vi "Read XML HW Configuration File_Parse Channels.vi"(8 "error in (no error)":errorcluster, 11 "channel429":refnum<k24>[](array[refnum])) -> (0 "error out":errorcluster, 3 "Array":T1[](array[typedef]) {"speed" items=["Auto", "Low", "High"]; "Labels"."scheduleBuildUnit" items=["Millisecond", "Microsecond"]})   [LabVIEW 2020]
doc: "This VI parses the XML HW DB."
uses:
  Controls/Ballard_Channel.ctl
  Controls/Ballard_Label.ctl
  Controls/Ballard_Word.ctl
  Controls/ARINCParam.ctl
  Shared/Controls and Global/TransferType.ctl
  Controls/Channel_direction.ctl
  Controls/Channel Speed.ctl
  C:/Users/NI/Desktop/GIT/Ballard-Arinc-429-Custom-Device/Source/System Explorer/SubVIs/Parse XML Ballard/Ballard_BTI_XML_Deserializer.dll
  Ballard_BTI_XML_Deserializer.dll
  Ballard Arinc-429 System Explorer.lvlib
  Shared/Ballard Arinc-429 Shared.lvlib
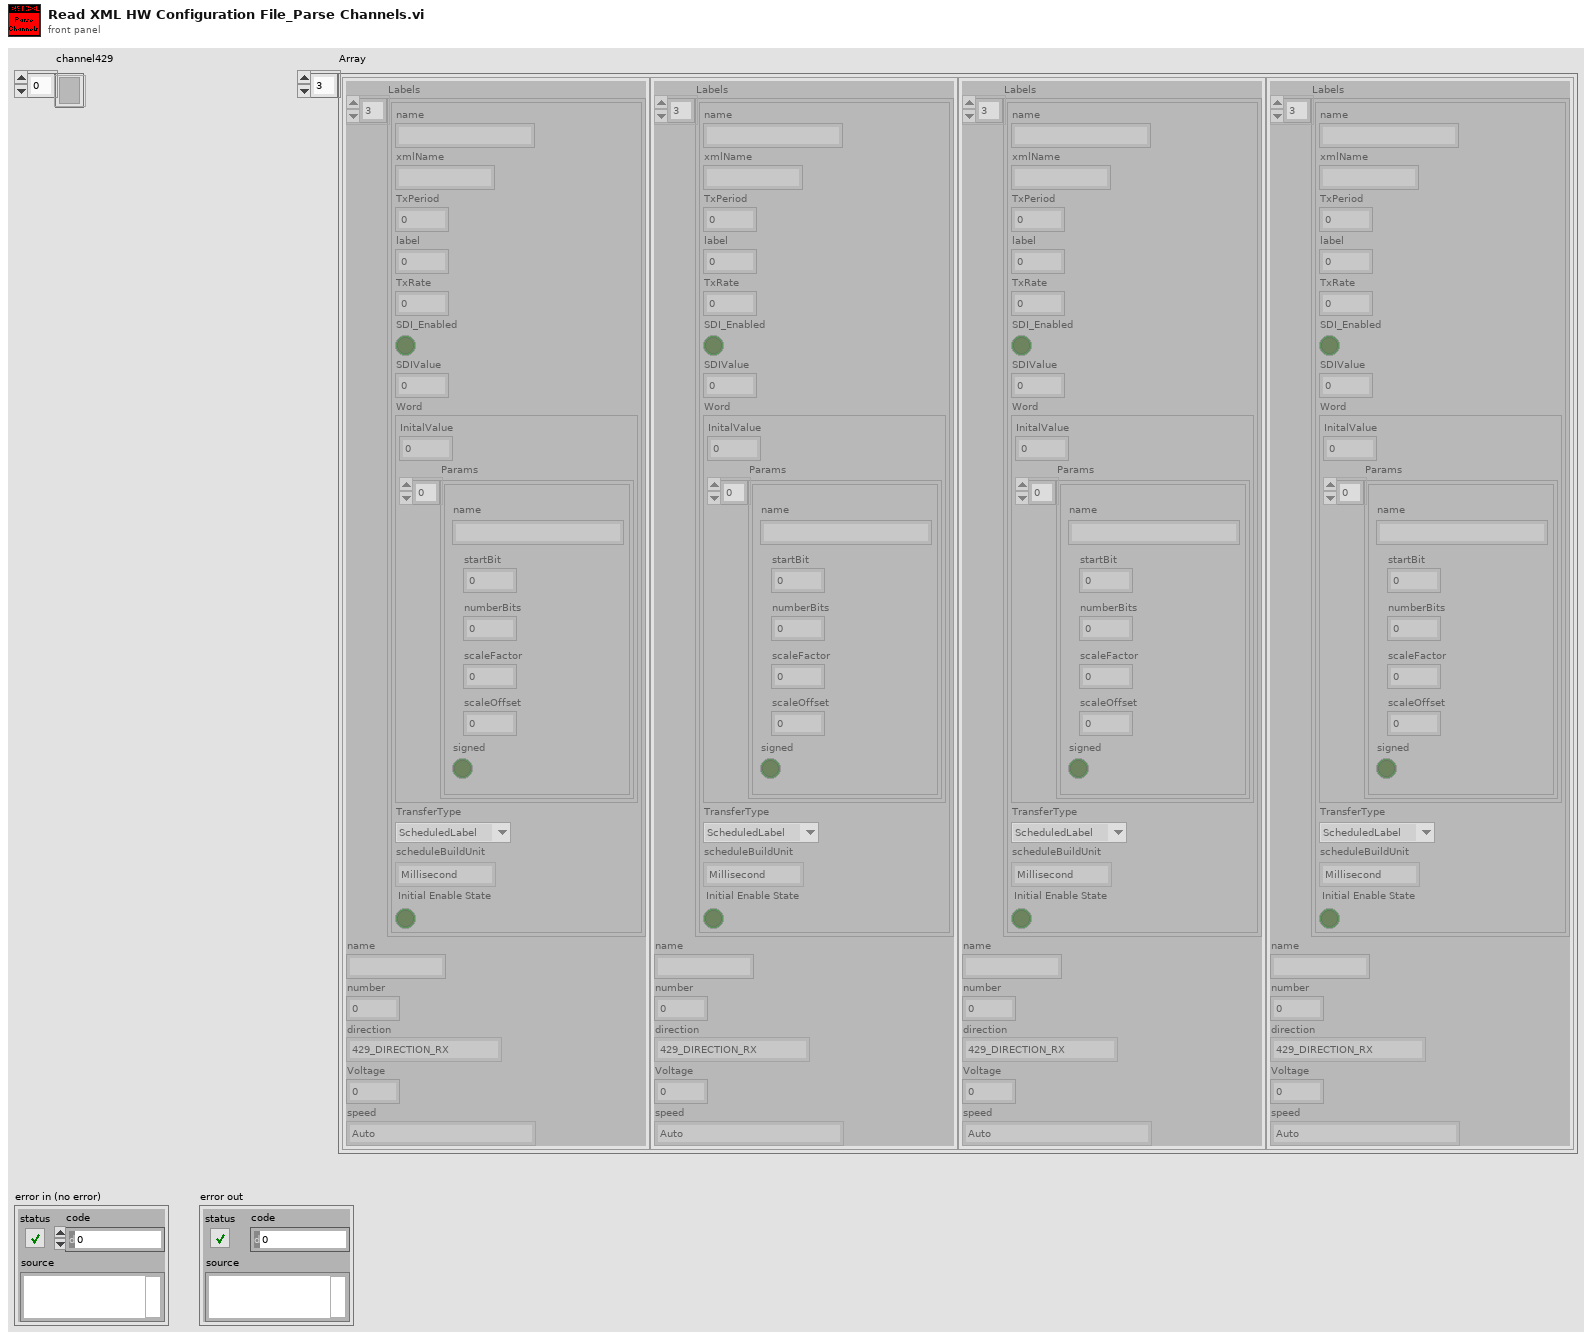
[diagram p1: front panel]
types:
  T1 = typedef "Ballard Arinc-429 System Explorer.lvlib/Ballard_Channel.ctl" = cluster{"Labels":T2[], "name":string, "number":u8, "direction":T6, "Voltage":dbl, "speed":T7}
  T2 = typedef "Ballard Arinc-429 System Explorer.lvlib/Ballard_Label.ctl" = cluster{"name":string, "xmlName":string, "TxPeriod":u32, "label":u32, "TxRate":dbl, "SDI_Enabled":bool, "SDIValue":u8, "Word":T3, "TransferType":T5, "scheduleBuildUnit":i32, "Initial Enable State":bool}
  T3 = typedef "Ballard Arinc-429 System Explorer.lvlib/Ballard_Word.ctl" = cluster{"InitalValue":u32, "Params":T4[]}
  T4 = typedef "Ballard Arinc-429 System Explorer.lvlib/ARINCParam.ctl" = cluster{"name":string, "startBit":i32, "numberBits":i32, "scaleFactor":dbl, "scaleOffset":dbl, "signed":bool}
  T5 = typedef "Ballard Arinc-429 Shared.lvlib/TransferType.ctl" = enum16{"ScheduledLabel", "Acyclic", "Block", "Strobe"}
  T6 = typedef "Ballard Arinc-429 System Explorer.lvlib/Channel_direction.ctl" = enum16{"429_DIRECTION_RX", "429_DIRECTION_TX"}
  T7 = typedef "Ballard Arinc-429 System Explorer.lvlib/Channel Speed.ctl" = i32
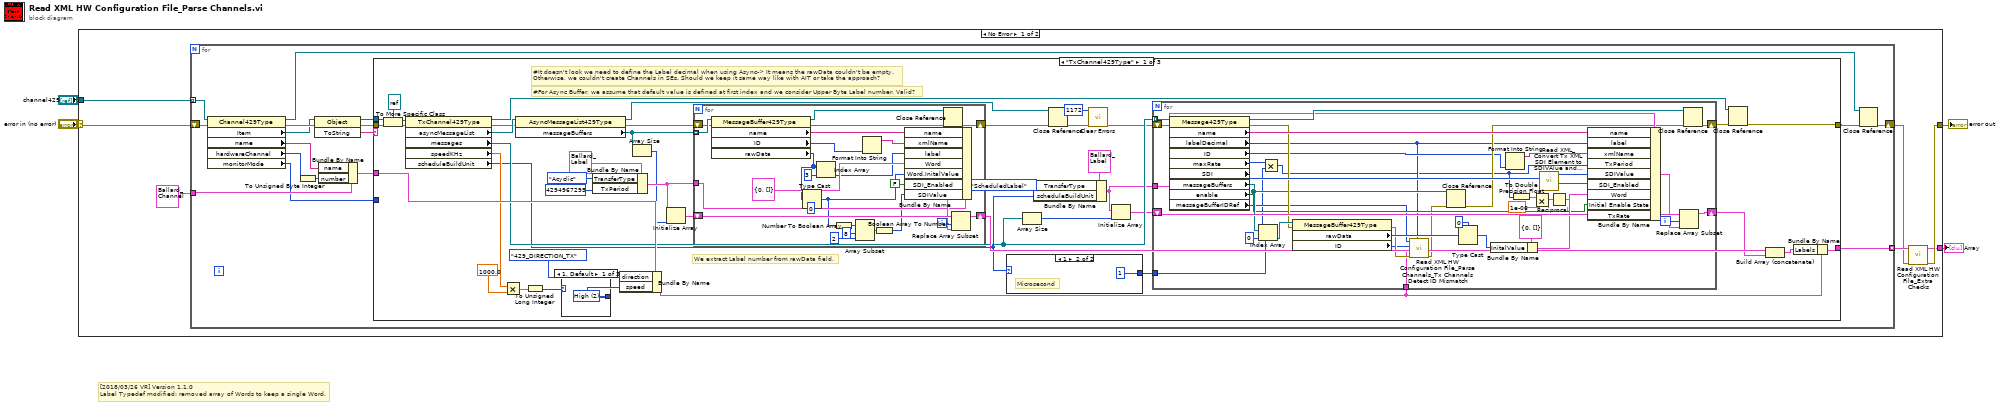
[diagram p0: block diagram]
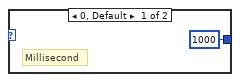
[diagram p2: hidden frame]
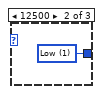
[diagram p3: hidden frame]
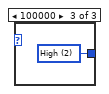
[diagram p4: hidden frame]
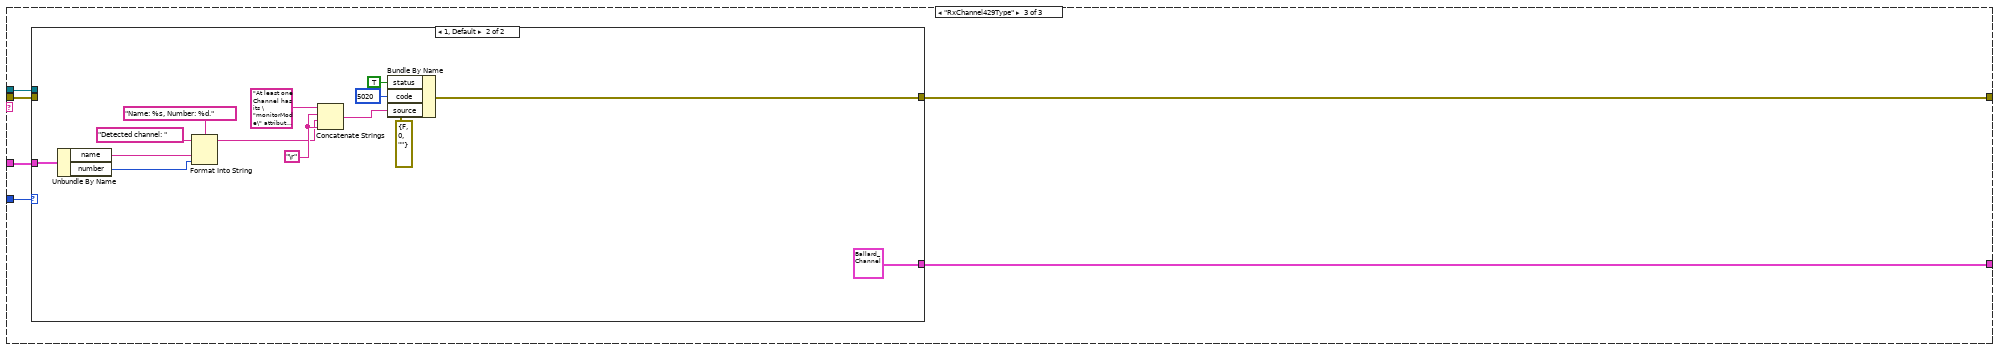
[diagram p6: hidden frame]
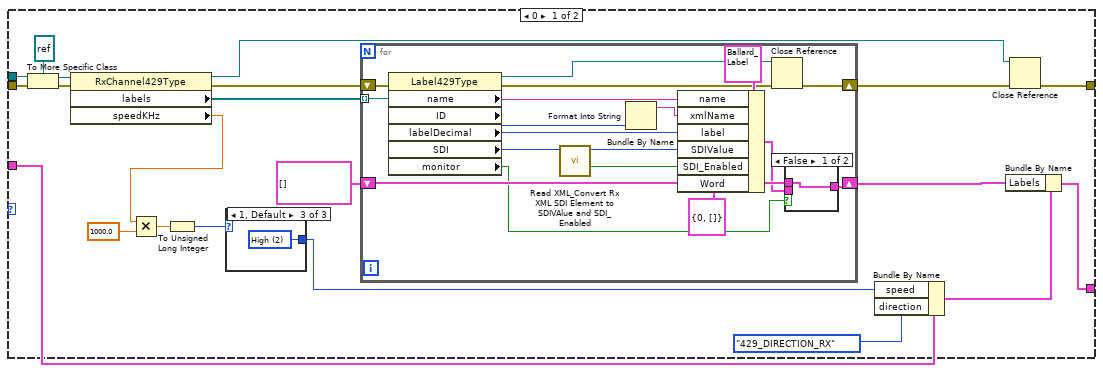
[diagram p7: hidden frame]
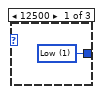
[diagram p8: hidden frame]
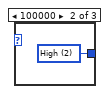
[diagram p9: hidden frame]
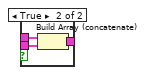
[diagram p10: hidden frame]
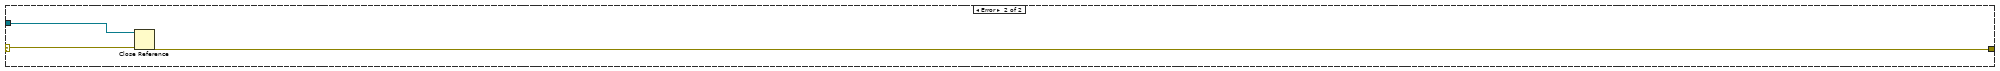
[diagram p11: hidden frame]
diagram:
  # "[2018/03/26 VR] Version 1.1.0\nLabel Typedef modified: removed array of Words to keep a single Word."
  n1 = case shown="No Error" "error in (no error)" {
    selector: "error in (no error)" -> [w9 w210]
    tunnel: [w5 _] -> w4
    tunnel: [w6 w209] -> w3
    tunnel: "channel429" -> [w10 w211]
    frame No Error {
      n2 = for {
        tunnel: w10 -> [w28] mode=indexing
        shift-right: [w16] -> w7
        shift-left: w9 -> [w25]
        tunnel: T1 {"Labels"=[], "name"="", "number"=0, "direction"=enum."429_DIRECTION_RX", "Voltage"=0.0, "speed"=0} ("channel") -> [w21]
        tunnel: [w12] -> w8 mode=indexing
        n3 = property class="Channel429Type"(reference=w28, error in=w25) -> (reference out=w15:refnum<k24>, error out=w24:errorcluster, "Item"=w22:refnum<k24>, "name"=w20:string, "hardwareChannel"=w19:i32, "monitorMode"=w14:i32)
        n4 = To Unsigned Byte Integer(number=w19) -> (unsigned 8bit integer=w18:u8)
        n5 = invoke class="Object" method="ToString"(reference=w22, error in=w24) -> (reference out=w26:refnum<k24>, error out=w23:errorcluster, "ToString"=w27:string)  [unwired: 1 in]
        n6 = Bundle By Name(cluster=w21, "name"=w20, "number"=w18) -> (w17:T1)
        n7 = case shown="\"TxChannel429Type\"" w27 {
          tunnel: w26 -> [w71 _ w148]
          tunnel: w23 -> [w70 w142 w147]
          tunnel: [w58 w142 w144] -> w13
          tunnel: w17 -> [w56 w141 w145]
          tunnel: [w45 w141 w146] -> w12
          tunnel: w14 -> [_ _ w143]
          frame "TxChannel429Type" {
            # "We extract Label number from rawData field."
            # "#For Async Buffer, we assume that default value is defined at first index and we consider Upper Byte Label number. Valid?"
            # "#It doesn't look we need to define the Label decimal when using Async-> It means the rawData couldn't be empty.\nOtherwise, we couldn't create Channels in SEs. Should we keep it same way like with AIT or take the approach?"
            n8 = To More Specific Class(target class=refnum<k24> refnum, reference=w71, error in=w70) -> (specific class reference=w67:refnum<k24>, error out=w68:errorcluster)
            n9 = property class="TxChannel429Type"(reference=w67, error in=w68) -> (reference out=w59:refnum<k24>, error out=w65:errorcluster, "asyncMessageList"=w66:refnum<k24>, "messages"=w43:refnum<k24>[], "speedKHz"=w38:dbl, "scheduleBuildUnit"=w30:i32)
            n10 = Multiply(x=w38, y=1000.0) -> (x*y=w39:dbl)
            n11 = property class="AsyncMessageList429Type"(reference=w66, error in=w65) -> (reference out=w61:refnum<k24>, error out=w64:errorcluster, "messageBuffers"=w52:refnum<k24>[])
            n12 = To Unsigned Long Integer(number=w39) -> (unsigned 32bit integer=w36:u32)
            n13 = case shown="1, Default" w36 {
              tunnel: [w74 w75 w76] -> w35
              frame 1, Default {
                w74 = T7 2 items=["Auto", "Low", "High"] ("speed")
              }
              frame 12500 {
                w75 = T7 1 items=["Auto", "Low", "High"] ("speed")
              }
              frame 100000 {
                w76 = T7 2 items=["Auto", "Low", "High"] ("speed")
              }
            }
            n14 = Bundle By Name(cluster=T2 {"name"="", "xmlName"="", "TxPeriod"=0, "label"=0, "TxRate"=0.0, "SDI_Enabled"=FALSE, "SDIValue"=0, "Word"={"InitalValue"=0, "Params"=[]}, "TransferType"=enum."ScheduledLabel", "scheduleBuildUnit"=0, "Initial Enable State"=FALSE} ("Label"), "TransferType"=TransferType."Acyclic", "TxPeriod"=u32 4294967295) -> (w53:T2)
            n15 = Bundle By Name(cluster=w56, "direction"=Channel_direction."429_DIRECTION_TX", "speed"=w35) -> (w31:T1)
            n16 = Array Size(array=w52) -> (size(s)=w51:i32)
            n17 = Initialize Array(w53, w51) -> (w50:T2[])
            n18 = for {
              tunnel: w52 -> [w140] mode=indexing
              shift-right: [w136] -> w63
              shift-left: w64 -> [w139]
              tunnel: w53 -> [w131]
              shift-right: [w134] -> w48
              shift-left: w50 -> [w135]
              i -> [w133]
              n19 = property class="MessageBuffer429Type"(reference=w140, error in=w139) -> (reference out=w137:refnum<k24>, error out=w138:errorcluster, "name"=w130:string, "ID"=w129:i32, "rawData"=w124:u8[])
              n20 = Type Cast(type=u32 0, x=w124) -> (*(type *) &x=w117:u32)
              n21 = Index Array(array=w124, index=3) -> (element=w123:u8)
              n22 = Number To Boolean Array(number=w117) -> (Boolean array=w118:bool[])
              n23 = Array Subset(array=w118, index=8, length=2) -> (w119:bool[])
              n24 = Format Into String(w129) -> (resulting string=w128:string)  [unwired: 3 in, 1 out]
              n25 = Boolean Array To Number(Boolean array=w119) -> (number=w116:u8)
              n26 = Bundle By Name(cluster=w131, "name"=w130, "xmlName"=w128, "label"=w123, "Word"=T3 {"InitalValue"=0, "Params"=[]}, "Word.InitalValue"=w117, "SDI_Enabled"=FALSE, "SDIValue"=w116) -> (w132:T2)
              n27 = Close Reference(reference=w137, error in (no error)=w138) -> (error out=w136:errorcluster)
              n28 = Replace Array Subset(array=w135, new element=w132, index=w133) -> (w134:T2[])
            }
            n29 = case shown="1" w30 {
              tunnel: [1000 1] -> w29
              frame 0, Default {
                # "Millisecond"
              }
              frame 1 {
                # "Microsecond"
              }
            }
            n30 = Array Size(array=w43) -> (size(s)=w41:i32)
            n31 = Bundle By Name(cluster=T2 {"name"="", "xmlName"="", "TxPeriod"=0, "label"=0, "TxRate"=0.0, "SDI_Enabled"=FALSE, "SDIValue"=0, "Word"={"InitalValue"=0, "Params"=[]}, "TransferType"=enum."ScheduledLabel", "scheduleBuildUnit"=0, "Initial Enable State"=FALSE} ("Label"), "TransferType"=TransferType."ScheduledLabel", "scheduleBuildUnit"=w30) -> (w42:T2)
            n32 = Close Reference(reference=w61, error in (no error)=w63) -> (error out=w62:errorcluster)
            n33 = call <vilib>:"Clear Errors.vi"("error in (no error)"=w62, "specific error code to clear (0: all)"=1172) -> ("error out"=w33:errorcluster)  [unwired: 4 in, 1 out]
            n34 = Initialize Array(w42, w41) -> (w40:T2[])
            n35 = for {
              tunnel: w43 -> [w115] mode=indexing
              shift-right: [w113] -> w60
              shift-left: w33 -> [w114]
              tunnel: w42 -> [w108]
              shift-right: [w111] -> w34
              shift-left: w40 -> [w109]
              tunnel: w31 -> [w86]
              tunnel: w29 -> [w82]
              i -> [w110]
              n36 = property class="Message429Type"(reference=w115, error in=w114) -> (reference out=w112:refnum<k24>, error out=w99:errorcluster, "name"=w107:string, "labelDecimal"=w84:i32, "ID"=w88:i32, "maxRate"=w83:i32, "SDI"=w104:i32, "messageBuffers"=w98:refnum<k24>[], "enable"=w91:bool, "messageBufferIDRef"=w85:i32)
              n37 = Index Array(array=w98, index=0) -> (element=w100:refnum<k24>)
              n38 = Multiply(x=w83, y=w82) -> (x*y=w81:i32)
              n39 = property class="MessageBuffer429Type"(reference=w100, error in=w99) -> (error out=w90:errorcluster, "rawData"=w93:u8[], "ID"=w87:i32)  [unwired: 1 out]
              n40 = call "Read XML HW Configuration File_Parse Channels_Tx Channels Detect ID Mismatch.vi"("Label"=w84, "error in (no error)"=w90, "channel"=w86, "messageBuffer ID"=w87, "messageBufferIDRef"=w85) -> ("error out"=w89:errorcluster)  [unwired: 6 in]
              n41 = Close Reference(reference=w98, error in (no error)=w89) -> (error out=w97:errorcluster)
              n42 = Type Cast(type=u32 0, x=w93) -> (*(type *) &x=w94:u32)
              n43 = Bundle By Name(cluster=T3 {"InitalValue"=0, "Params"=[]} ("Word"), "InitalValue"=w94) -> (w92:T3)
              n44 = Format Into String(w88) -> (resulting string=w105:string)  [unwired: 3 in, 1 out]
              n45 = To Double Precision Float(number=w81) -> (double precision float=w80:dbl)
              n46 = Multiply(x=w80, y=1e-06) -> (x*y=w78:dbl)
              n47 = call "Read XML_Convert Tx XML SDI Element to SDIVAlue and SDI_Enabled.vi"("SDI"=w104) -> ("SDI_Enabled"=w102:bool, "SDIValue"=w103:u8)  [unwired: 9 in]
              n48 = Reciprocal(x=w78) -> (1/x=w77:dbl)
              n49 = Bundle By Name(cluster=w108, "name"=w107, "label"=w84, "xmlName"=w105, "TxPeriod"=w81, "SDIValue"=w103, "SDI_Enabled"=w102, "Word"=w92, "Initial Enable State"=w91, "TxRate"=w77) -> (w106:T2)
              n50 = Replace Array Subset(array=w109, new element=w106, index=w110) -> (w111:T2[])
              n51 = Close Reference(reference=w112, error in (no error)=w97) -> (error out=w113:errorcluster)
            }
            n52 = Close Reference(reference=w59, error in (no error)=w60) -> (error out=w58:errorcluster)
            n53 = Build Array (concatenate)(w48, w34) -> (w44:T2[])
            n54 = Bundle By Name(cluster=w31, "Labels"=w44) -> (w45:T1)
          }
          frame "False", Default {
          }
          frame "RxChannel429Type" {
            n55 = case shown="1, Default" w143 {
              tunnel: w148 -> [w169 _]
              tunnel: w147 -> [w168 _]
              tunnel: [w160 T1 {"Labels"=[], "name"="", "number"=0, "direction"=enum."429_DIRECTION_RX", "Voltage"=0.0, "speed"=0} ("channel")] -> w146
              tunnel: w145 -> [w158 w200]
              tunnel: [w155 w204] -> w144
              frame 0 {
                n56 = To More Specific Class(target class=refnum<k24> refnum, reference=w169, error in=w168) -> (specific class reference=w165:refnum<k24>, error out=w166:errorcluster)
                n57 = property class="RxChannel429Type"(reference=w165, error in=w166) -> (reference out=w154:refnum<k24>, error out=w163:errorcluster, "labels"=w164:refnum<k24>[], "speedKHz"=w151:dbl)
                n58 = Multiply(x=w151, y=1000.0) -> (x*y=w153:dbl)
                n59 = To Unsigned Long Integer(number=w153) -> (unsigned 32bit integer=w150:u32)
                n60 = case shown="1, Default" w150 {
                  tunnel: [w170 w171 w172] -> w149
                  frame 12500 {
                    w170 = T7 1 items=["Auto", "Low", "High"] ("speed")
                  }
                  frame 100000 {
                    w171 = T7 2 items=["Auto", "Low", "High"] ("speed")
                  }
                  frame 1, Default {
                    w172 = T7 2 items=["Auto", "Low", "High"] ("speed")
                  }
                }
                n61 = for {
                  tunnel: w164 -> [w190] mode=indexing
                  shift-right: [w179] -> w156
                  shift-left: w163 -> [w189]
                  shift-right: [w187] -> w159
                  shift-left: T2[] [] ("Labels") -> [w188]
                  n62 = property class="Label429Type"(reference=w190, error in=w189) -> (reference out=w178:refnum<k24>, error out=w180:errorcluster, "name"=w182:string, "ID"=w183:i32, "labelDecimal"=w185:i32, "SDI"=w177:i32, "monitor"=w174:bool)
                  n63 = call "Read XML_Convert Rx XML SDI Element to SDIVAlue and SDI_Enabled.vi"("SDI"=w177) -> ("SDI_Enabled"=w175:bool, "SDIValue"=w176:u8)  [unwired: 9 in]
                  n64 = Format Into String(w183) -> (resulting string=w184:string)  [unwired: 3 in, 1 out]
                  n65 = Bundle By Name(cluster=T2 {"name"="", "xmlName"="", "TxPeriod"=0, "label"=0, "TxRate"=0.0, "SDI_Enabled"=FALSE, "SDIValue"=0, "Word"={"InitalValue"=0, "Params"=[]}, "TransferType"=enum."ScheduledLabel", "scheduleBuildUnit"=0, "Initial Enable State"=FALSE} ("TxScheduledLabel"), "name"=w182, "xmlName"=w184, "label"=w185, "SDIValue"=w176, "SDI_Enabled"=w175, "Word"=T3 {"InitalValue"=0, "Params"=[]}) -> (w181:T2)
                  n66 = Close Reference(reference=w178, error in (no error)=w180) -> (error out=w179:errorcluster)
                  n67 = case shown="False" w174 {
                    tunnel: w188 -> [w191 w194]
                    tunnel: [w191 w193] -> w187
                    tunnel: w181 -> [_ w192]
                    frame False {
                    }
                    frame True {
                      n68 = Build Array (concatenate)(w194, w192) -> (w193:T2[])
                    }
                  }
                }
                n69 = Bundle By Name(cluster=w158, "speed"=w149, "direction"=Channel_direction."429_DIRECTION_RX") -> (w161:T1)
                n70 = Bundle By Name(cluster=w161, "Labels"=w159) -> (w160:T1)
                n71 = Close Reference(reference=w154, error in (no error)=w156) -> (error out=w155:errorcluster)
              }
              frame 1, Default {
                w199 = "\r"
                n72 = Unbundle By Name(w200) -> ("name"=w198:string, "number"=w197:u8)
                n73 = Format Into String(format string="Name: %s, Number: %d.", initial string="Detected channel: ", w198, w197) -> (resulting string=w196:string)  [unwired: 1 in, 1 out]
                n74 = Concatenate Strings("At least one Channel has its \"monitorMode\" attribute set to \"All\" which is not supported. Only \"Selective\" value (default value) is supported for this attribute.", w199, w196, w199) -> (w205:string)
                n75 = Bundle By Name(cluster=errorcluster {"status"=FALSE, "code"=0, "source"=""} ("error in (no error) 2"), "status"=TRUE, "code"=5020, "source"=w205) -> (w204:errorcluster)
              }
            }
          }
        }
        n76 = Close Reference(reference=w15, error in (no error)=w13) -> (error out=w16:errorcluster)
      }
      n77 = call "Read XML HW Configuration File_Extra Checks.vi"("error in (no error)"=w7, "Array In"=w8) -> ("error out"=w6:errorcluster, "Array Out"=w5:T1[])  [unwired: 8 in]
    }
    frame Error {
      n78 = Close Reference(reference=w211, error in (no error)=w210) -> (error out=w209:errorcluster)
    }
  }
  "Array" <- w4
  "error out" <- w3
